vi "Single Relay Set.vi"(8 "error in (no error)":errorcluster, 9 "Relay No":i32, 10 "ON/OFF":bool, 11 "VISA resource name":refnum<visa-resource-name>) -> (0 "error out":errorcluster, 3 "VISA resource name out":refnum<visa-resource-name>)   [LabVIEW 2023, in "Numato.lvlib"]
uses:
  Numato.lvlib
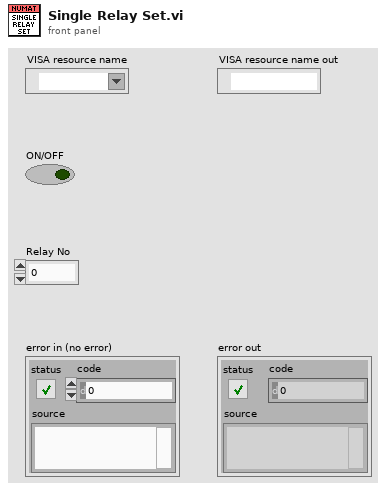
[diagram p1: front panel]
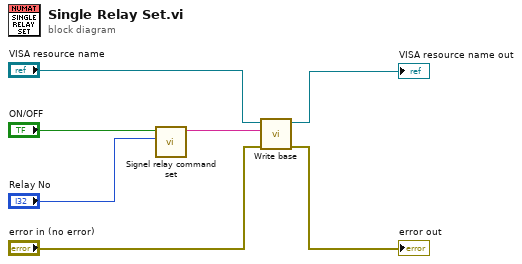
[diagram p0: block diagram]
diagram:
  n1 = call "Signel relay command set.vi"("Relay No"="Relay No", "ON/OFF"="ON/OFF") -> ("Command"=w2:string)  [unwired: 9 in]
  n2 = call "Write base.vi"("error in (no error)"="error in (no error)", "Command"=w2, "VISA resource name"="VISA resource name") -> ("error out"=→"error out":errorcluster, "VISA resource name out"=→"VISA resource name out":refnum<visa-resource-name>)  [unwired: 7 in]
